vi "hidden_deltas.vi"(9 "Forward Delta":dbl[](array[numeric]), 10 "Forward Weights":dbl[][](array[numeric]), 11 "Node Outputs":dbl[](array[numeric])) -> (3 "Current delta":dbl[](array[numeric]))   [LabVIEW 2018]
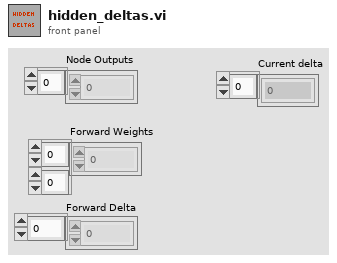
[diagram p1: front panel]
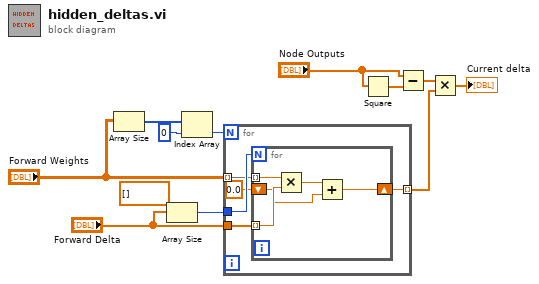
[diagram p0: block diagram]
diagram:
  (unwired) dbl[] []
  n1 = Array Size(array="Forward Weights") -> (size(s)=w7:i32[])
  n2 = Array Size(array="Forward Delta") -> (size(s)=w4:i32)
  n3 = Index Array(array=w7, index=0) -> (element=w5:i32)
  n4 = for {
    N: w5 -> [_]
    tunnel: w4 -> [w16]
    tunnel: "Forward Delta" -> [w15]
    tunnel: "Forward Weights" -> [w14] mode=indexing
    tunnel: [w12] -> w1 mode=indexing
    n5 = for {
      N: w16 -> [_]
      tunnel: w15 -> [w21] mode=indexing
      tunnel: w14 -> [w20] mode=indexing
      shift-right: [w18] -> w12
      shift-left: 0.0 -> [w17]
      n6 = Multiply(x=w20, y=w21) -> (x*y=w19:dbl)
      n7 = Add(x=w19, y=w17) -> (x+y=w18:dbl)
    }
  }
  n8 = Square(x="Node Outputs") -> (x^2=w10:dbl[])
  n9 = Subtract(x="Node Outputs", y=w10) -> (x-y=w9:dbl[])
  n10 = Multiply(x=w9, y=w1) -> (x*y=→"Current delta":dbl[])
